vi "Rasnik_SAVE.vi"() -> ()   [LabVIEW 2015]
uses:
  GlobalPath.vi
  Desktop/Mari/GlobalData.vi
panel:
  out "Script":path
  out "Logfile Path":path
  out "Filename selected":path
  out "standard output":string
  out "Y D10":dbl format="%.2f"
  out "Y D9":dbl format="%.2f"
  out "Y D8":dbl format="%.2f"
  out "Y D7":dbl format="%.2f"
  out "Y D6":dbl format="%.2f"
  out "Y D5":dbl format="%.2f"
  out "Y D4":dbl format="%.2f"
  out "Y D3":dbl format="%.2f"
  out "Y D2":dbl format="%.2f"
  out "Y D1":dbl format="%.2f"
  out "X D10":dbl format="%.2f"
  out "X D9":dbl format="%.2f"
  out "X D8":dbl format="%.2f"
  out "X D7":dbl format="%.2f"
  out "X D6":dbl format="%.2f"
  out "X D5":dbl format="%.2f"
  out "X D4":dbl format="%.2f"
  out "X D3":dbl format="%.2f"
  out "X D2":dbl format="%.2f"
  out "X D1":dbl format="%.2f"
  out "Latest file: 2":path
  out "y 6":string
  out "x 6":string
  in  "Done?":bool
  out "y 10":string
  out "x 10":string
  out "y 9":string
  out "x 9":string
  out "y 8":string
  out "x 8":string
  out "y 7":string
  out "x 7":string
  out "y 5":string
  out "x 5":string
  out "y 4":string
  out "x 4":string
  out "y 3":string
  out "x 3":string
  out "y 2":string
  out "x 2":string
  out "y 1":string
  out "x 1":string
  out "Lines":string[](array[string])
  out "Latest file:":path
  in  "Open Program":bool
  in  "c-ccd 3":bool caption="Setup the electronics for the C-CCD reading:\n- make sure the ethernet cables are connected on the minimal heads\n- check that the cable connecting the driver with the mux is plugged in\n- verify that the driver is on and connected to the LAN"
  in  "c-ccd":bool caption="Read the data file"
  # "Rasmask reading from PCBs on stiffback/table"
  # "Run the C-CCD reading program \n(the 10 Rasmasks are automatically read and the data saved)"
  # "Data file reading"
  # "The most recent data file created by the C-CCD program will be opened.\nOnce the \"read data file\" is clicked, the raw data and displacement should appear on the PCB schematics on the bottom."
  # "Displacement (um):"
  # "Raw Data (um):"
  # "Rasmask 1"
  # "Rasmask 2"
  # "Rasmask 1"
  # "Rasmask 2"
  # "Rasmask 3"
  # "Rasmask 4"
  # "Rasmask 3"
  # "Rasmask 4"
  # "Rasmask 6"
  # "Rasmask 5"
  # "Rasmask 6"
  # "Rasmask 5"
  # "Rasmask 7"
  # "Rasmask 8"
  # "Rasmask 7"
  # "Rasmask 8"
  # "Rasmask 9"
  # "Rasmask 10"
  # "Rasmask 9"
  # "Rasmask 10"
  # "Open the DB and load the Rarnik raw file:\nClick on the tab \"RO measurement\" and on the bottom click on \"Load Rasnik 1\" for the table and \"Load  Rasnik 2\" for the stiffback\nLoad the file that appears here --------------------------------------------------------------->\nPress \"SAve info to database\""
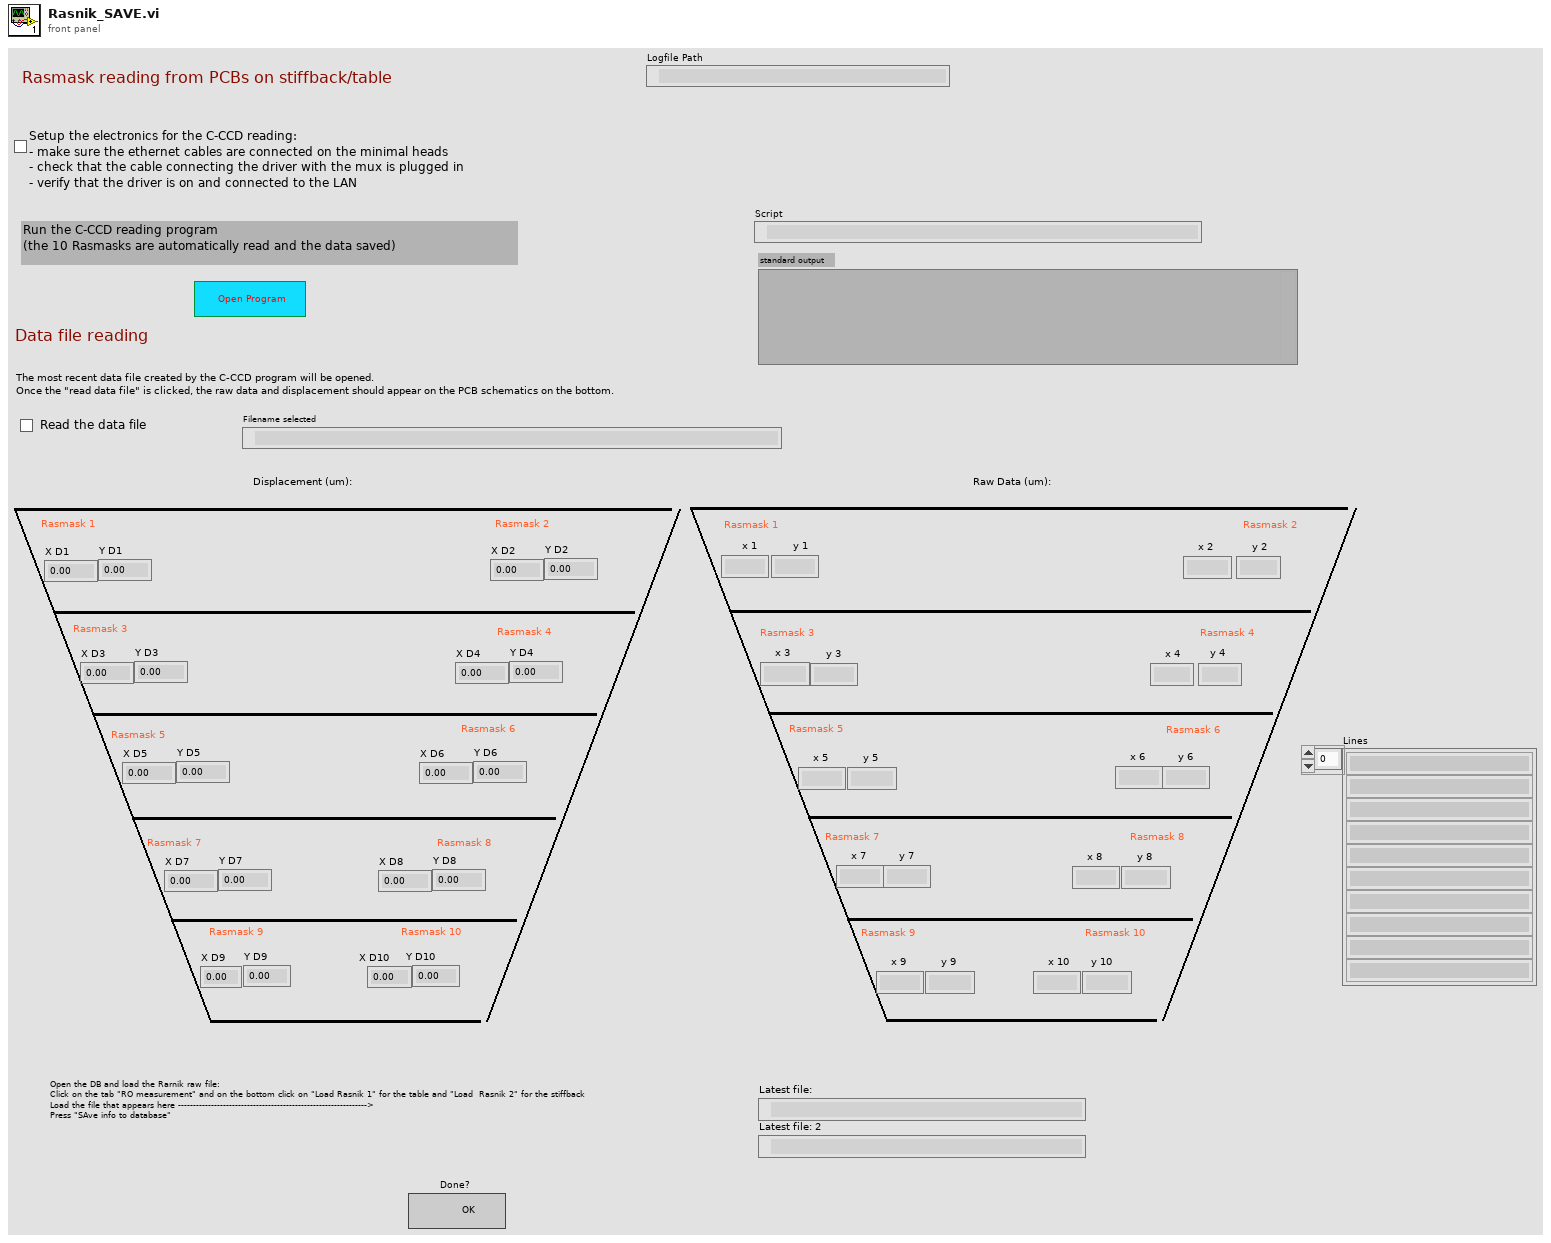
[diagram p1: front panel]
types:
  T1 = enum16{"open", "replace", "create", "open or create", "replace or create", "replace or create with confirmation"}
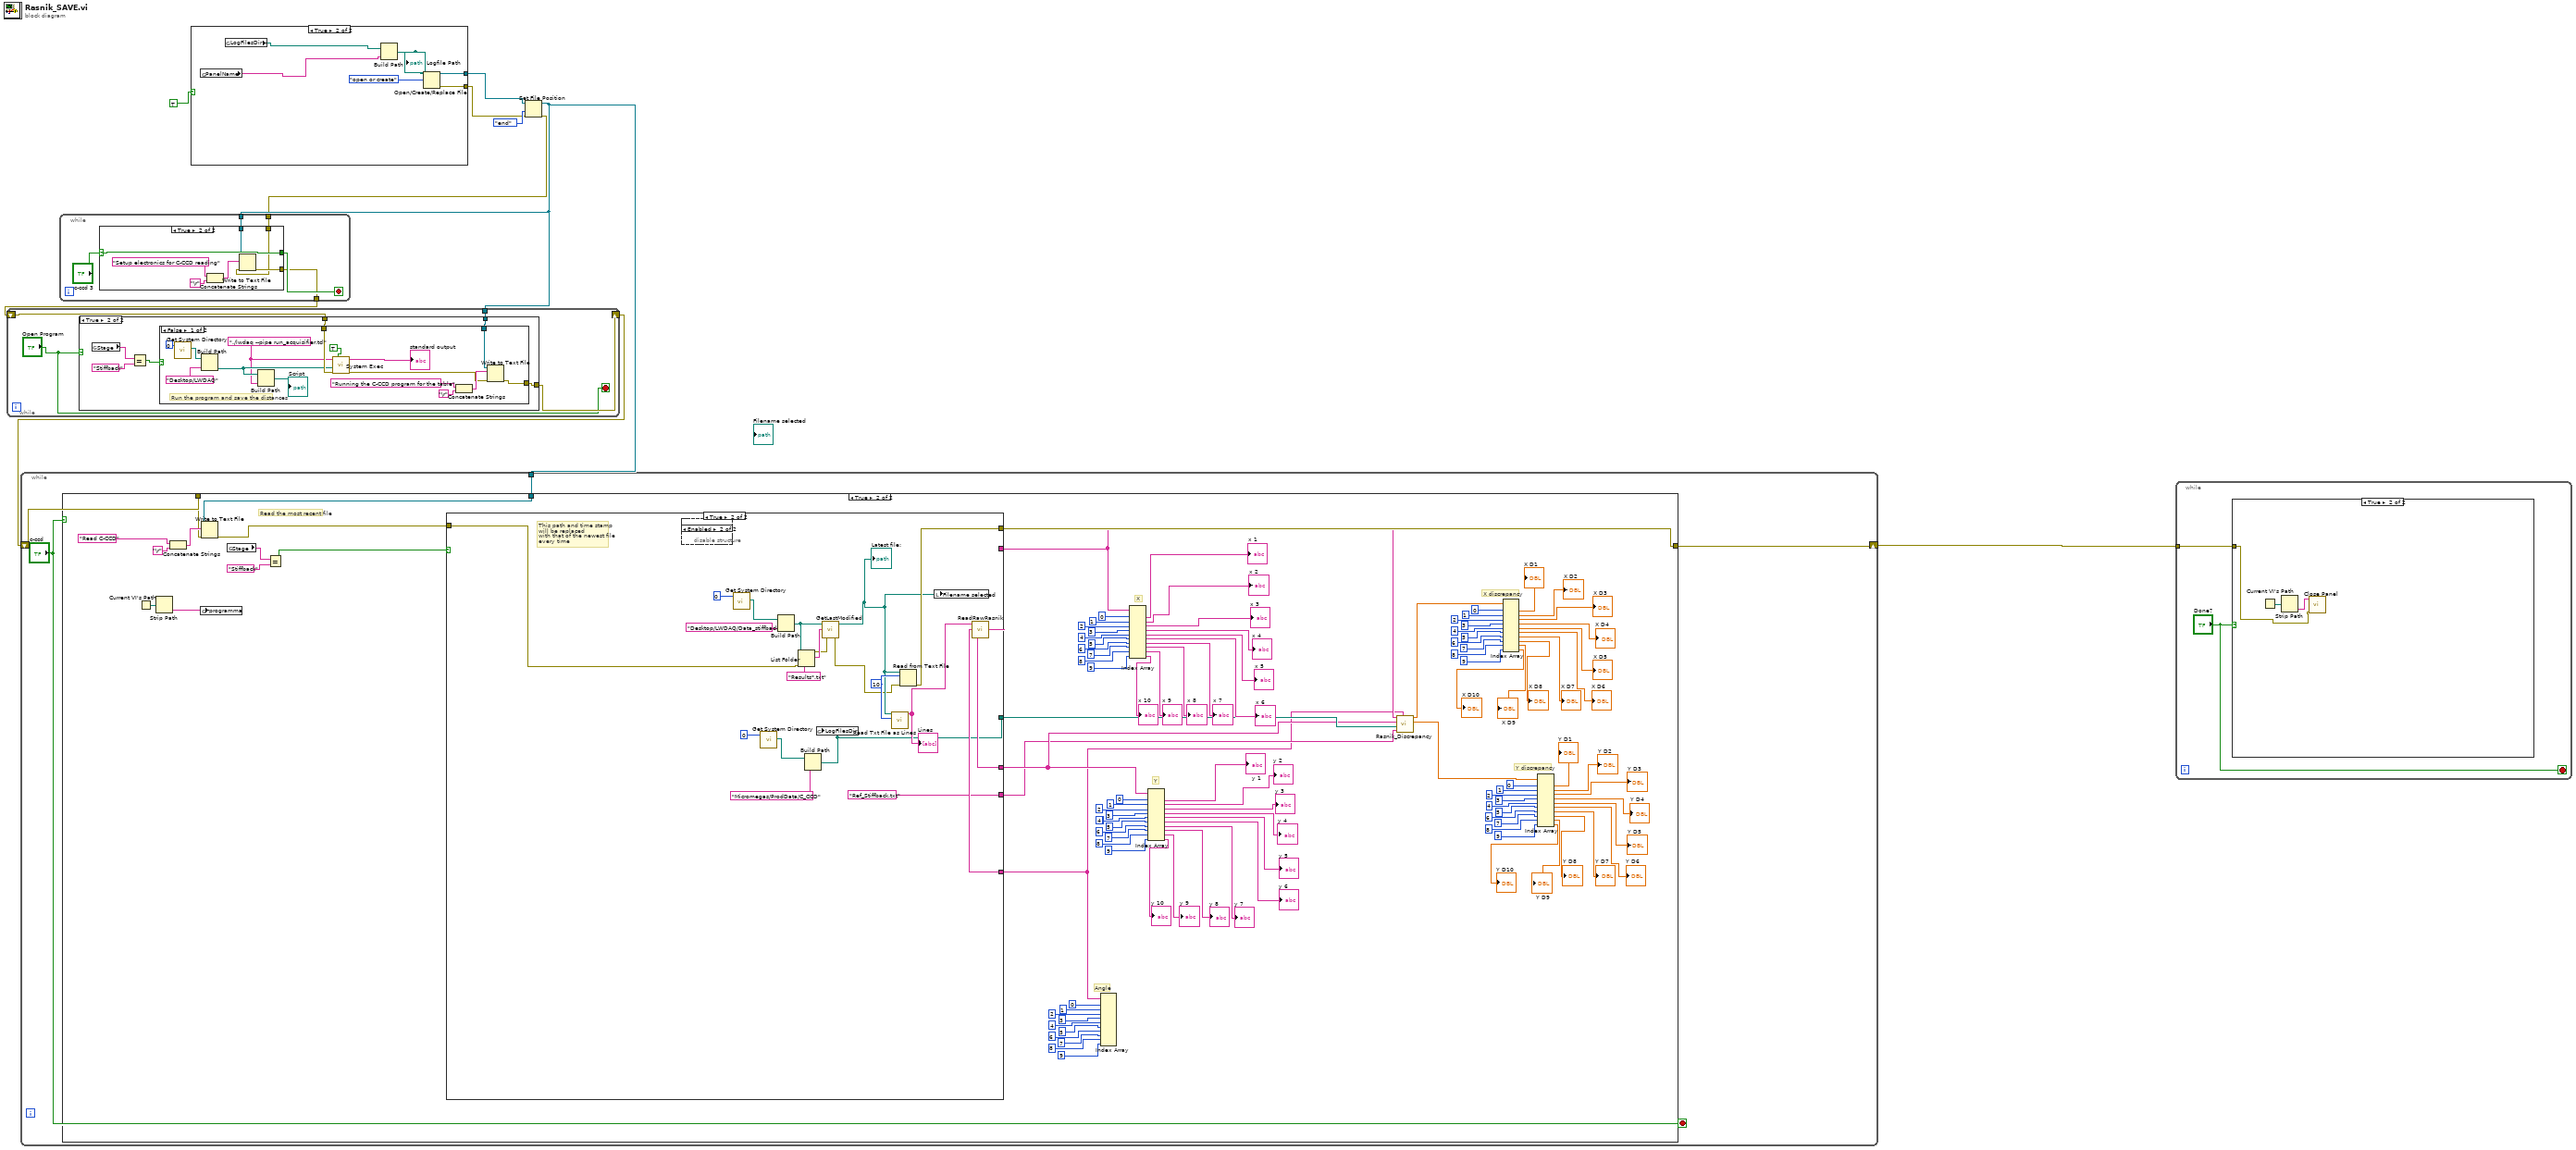
[diagram p0: block diagram]
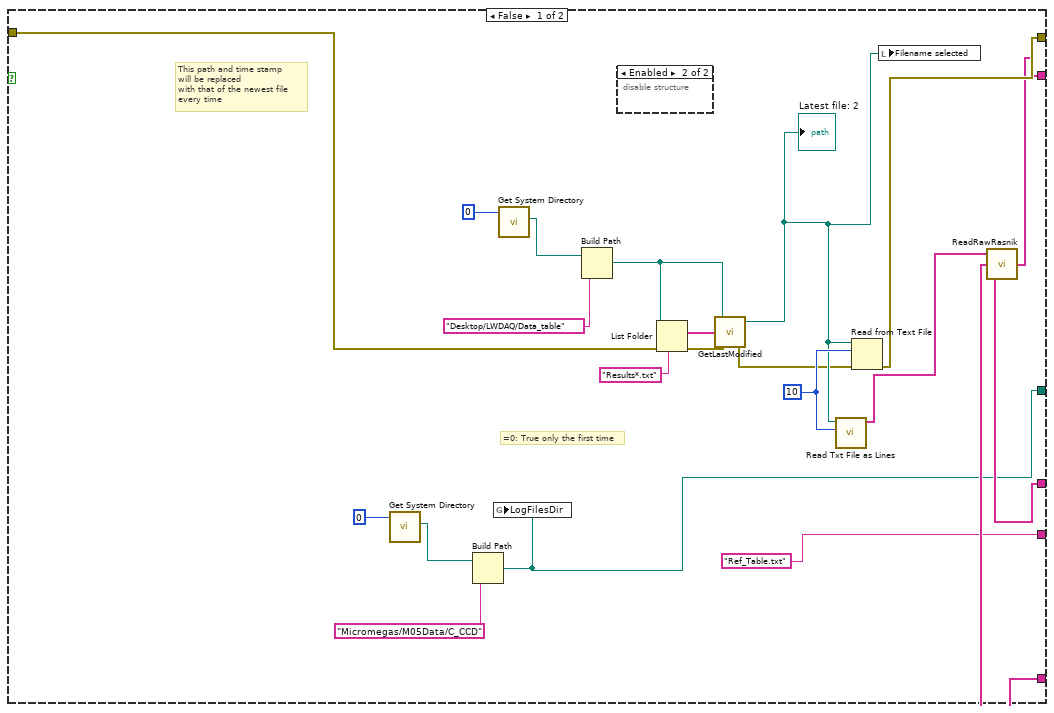
[diagram p4: hidden frame]
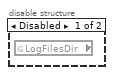
[diagram p5: hidden frame]
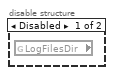
[diagram p6: hidden frame]
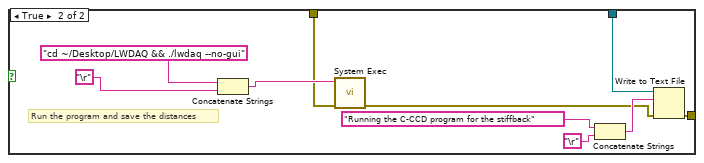
[diagram p9: hidden frame]
diagram:
  n1 = case shown="True" TRUE {
    tunnel: [_ w14] -> w3
    tunnel: [_ w13] -> w4
    frame False {
    }
    frame True {
      n2 = global read "GlobalData.vi" "PanelName"() -> (w10:string)
      n3 = global read "GlobalPath.vi" "LogFilesDir"() -> (w11:path)
      n4 = Build Path(base path=w11, name or relative path=w10) -> (appended path=w15:path)
      "Logfile Path" <- w15
      n5 = Open/Create/Replace File(file path (use dialog)=w15, operation (0:open)=T1."open or create") -> (refnum out=w14:refnum<file>, error out=w13:errorcluster)  [unwired: 4 in, 1 out]
    }
  }
  n6 = Set File Position(refnum=w3, from (0:start)=enum16{"start", "end", "current"}."end", error in=w4) -> (refnum out=w2:refnum<file>, error out=w1:errorcluster)  [unwired: 1 in]
  n7 = while {
    tunnel: w2 -> [w19]
    tunnel: [w17] -> w7
    tunnel: w1 -> [w16]
    stop <- w18 stop-if-true
    n8 = case shown="True" "c-ccd 3" {
      selector: "c-ccd 3" -> [_ w23]
      tunnel: [_ w24] -> w17
      tunnel: w19 -> [_ w21]
      tunnel: [_ w23] -> w18
      tunnel: w16 -> [_ w22]
      frame False {
      }
      frame True {
        n9 = Concatenate Strings("Setup electronics for C-CCD reading", "\r") -> (w27:string)
        n10 = Write to Text File(file (use dialog)=w21, text=w27, error in=w22) -> (error out=w24:errorcluster)  [unwired: 1 in, 2 out]
      }
    }
  }
  n11 = while {
    tunnel: w2 -> [w29]
    shift-right: [w30] -> w9
    shift-left: w7 -> [w31]
    stop <- "Open Program" stop-if-true
    n12 = case shown="True" "Open Program" {
      tunnel: w31 -> [w32 w35]
      tunnel: [w32 w34] -> w30
      tunnel: w29 -> [_ w33]
      frame False {
      }
      frame True {
        n13 = global read "GlobalData.vi" "Stage"() -> (w37:string)
        n14 = Equal?(x=w37, y="Stiffback") -> (x = y?=w36:bool)
        n15 = case shown="False" w36 {
          tunnel: w35 -> [w50 w57]
          tunnel: [w48 w55] -> w34
          tunnel: w33 -> [w47 w54]
          frame False {
            w40 = "./lwdaq --pipe run_acquisifier.tcl"
            # "Run the program and save the distances"
            n16 = call <vilib>:"Get System Directory.vi"("system directory type"=0) -> ("system directory"=w45:path)  [unwired: 10 in]
            n17 = Build Path(base path=w45, name or relative path="Desktop/LWDAQ") -> (appended path=w41:path)
            n18 = Build Path(base path=w41, name or relative path=w40) -> (appended path=→"Script":path)
            n19 = call <vilib>:"System Exec.vi"("wait until completion? (T)"=TRUE, "error in (no error)"=w50, "working directory"=w41, "command line"=w40) -> ("error out"=w49:errorcluster, "standard output"=→"standard output":string)  [unwired: 4 in, 2 out]
            n20 = Concatenate Strings("Running the C-CCD program for the table", "\r") -> (w53:string)
            n21 = Write to Text File(file (use dialog)=w47, text=w53, error in=w49) -> (error out=w48:errorcluster)  [unwired: 1 in, 2 out]
          }
          frame True {
            # "Run the program and save the distances"
            n22 = Concatenate Strings("cd ~/Desktop/LWDAQ && ./lwdaq --no-gui", "\r") -> (w62:string)
            n23 = call <vilib>:"System Exec.vi"("error in (no error)"=w57, "command line"=w62) -> ("error out"=w56:errorcluster)  [unwired: 6 in, 3 out]
            n24 = Concatenate Strings("Running the C-CCD program for the stiffback", "\r") -> (w60:string)
            n25 = Write to Text File(file (use dialog)=w54, text=w60, error in=w56) -> (error out=w55:errorcluster)  [unwired: 1 in, 2 out]
          }
        }
      }
    }
  }
  n26 = while {
    tunnel: w2 -> [w65]
    shift-right: [w66] -> w8
    shift-left: w9 -> [w67]
    stop <- "c-ccd" stop-if-true
    n27 = case shown="True" "c-ccd" {
      tunnel: w67 -> [w68 w169]
      tunnel: [w68 w167] -> w66
      tunnel: w65 -> [_ w166]
      frame False {
      }
      frame True {
        (unwired) 6
        (unwired) 4
        (unwired) 3
        # "Y discrepancy"
        # "X discrepancy"
        # "Angle"
        # "Y"
        # "X"
        # "Read the most recent file"
        n28 = Current VI's Path() -> (path=w170:path)
        n29 = Strip Path(path=w170) -> (name=w171:string)  [unwired: 1 out]
        n30 = Concatenate Strings("Read C-CCD", "\r") -> (w177:string)
        n31 = global write "GlobalData.vi" "programma"(w171) -> ()
        n32 = Write to Text File(file (use dialog)=w166, text=w177, error in=w169) -> (error out=w168:errorcluster)  [unwired: 1 in, 2 out]
        n33 = global read "GlobalData.vi" "Stage"() -> (w173:string)
        n34 = Equal?(x=w173, y="Stiffback") -> (x = y?=w172:bool)
        n35 = case shown="True" w172 {
          tunnel: w168 -> [w178 w199]
          tunnel: [w195 w217] -> w167
          tunnel: [w194 w216] -> w114
          tunnel: [w196 w215] -> w113
          tunnel: [w193 w214] -> w69
          tunnel: [w185 w205] -> w115
          tunnel: ["Ref_Table.txt" "Ref_Stiffback.txt"] -> w112
          frame False {
            w198 = 10
            # "=0: True only the first time"
            # "This path and time stamp\nwill be replaced\nwith that of the newest file \nevery time"
            n36 = call <vilib>:"Get System Directory.vi"("system directory type"=0) -> ("system directory"=w187:path)  [unwired: 10 in]
            n37 = Build Path(base path=w187, name or relative path="Micromegas/M05Data/C_CCD") -> (appended path=w185:path)
            n38 = global write "GlobalPath.vi" "LogFilesDir"(w185) -> ()
            n39 = call <vilib>:"Get System Directory.vi"("system directory type"=0) -> ("system directory"=w190:path)  [unwired: 10 in]
            n40 = Build Path(base path=w190, name or relative path="Desktop/LWDAQ/Data_table") -> (appended path=w180:path)
            n41 = disable-structure shown="Enabled" {
              frame Disabled {
                n42 = global read "GlobalPath.vi" "LogFilesDir"() -> ()  [unwired: 1 out]
              }
              frame Enabled {
              }
            }
            n43 = List Folder(path=w180, pattern="Results*.txt", error in=w178) -> (filenames=w184:string[], error out=w181:errorcluster)  [unwired: 1 in, 2 out]
            n44 = call "GetLastModified.vi"("error in"=w181, "filenames"=w184, "SearchDir"=w180) -> ("error out"=w182:errorcluster, "Path"=w183:path)  [unwired: 1 out]
            "Latest file: 2" <- w183
            n45 = call "Read Txt File as Lines.vi"("Lines to Read"=w198, "file path (use dialog)"=w183) -> ("Lines"=w197:string[])  [unwired: 8 in, 1 out]
            n46 = Read from Text File(file (use dialog)=w183, count=w198, error in=w182) -> (error out=w195:errorcluster)  [unwired: 1 in, 3 out]
            n47 = local write "Filename selected"(w183) -> ()
            n48 = call "ReadRawRasnik.vi"("Lines"=w197) -> ("X cluster"=w194:string[], "Y cluster"=w196:string[], "angle cluster"=w193:string[])
          }
          frame True {
            w219 = 10
            # "This path and time stamp\nwill be replaced\nwith that of the newest file \nevery time"
            n49 = disable-structure shown="Enabled" {
              frame Disabled {
                n50 = global read "GlobalPath.vi" "LogFilesDir"() -> ()  [unwired: 1 out]
              }
              frame Enabled {
              }
            }
            n51 = call <vilib>:"Get System Directory.vi"("system directory type"=0) -> ("system directory"=w211:path)  [unwired: 10 in]
            n52 = call <vilib>:"Get System Directory.vi"("system directory type"=0) -> ("system directory"=w207:path)  [unwired: 10 in]
            n53 = Build Path(base path=w211, name or relative path="Desktop/LWDAQ/Data_stiffback") -> (appended path=w202:path)
            n54 = List Folder(path=w202, pattern="Results*.txt", error in=w199) -> (filenames=w201:string[], error out=w200:errorcluster)  [unwired: 1 in, 2 out]
            n55 = Build Path(base path=w207, name or relative path="Micromegas/ProdData/C_CCD") -> (appended path=w205:path)
            n56 = global write "GlobalPath.vi" "LogFilesDir"(w205) -> ()
            n57 = call "GetLastModified.vi"("error in"=w200, "filenames"=w201, "SearchDir"=w202) -> ("error out"=w203:errorcluster, "Path"=w204:path)  [unwired: 1 out]
            "Latest file:" <- w204
            n58 = call "Read Txt File as Lines.vi"("Lines to Read"=w219, "file path (use dialog)"=w204) -> ("Lines"=w218:string[])  [unwired: 8 in, 1 out]
            "Lines" <- w218
            n59 = Read from Text File(file (use dialog)=w204, count=w219, error in=w203) -> (error out=w217:errorcluster)  [unwired: 1 in, 3 out]
            n60 = local write "Filename selected"(w204) -> ()
            n61 = call "ReadRawRasnik.vi"("Lines"=w218) -> ("X cluster"=w216:string[], "Y cluster"=w215:string[], "angle cluster"=w214:string[])
          }
        }
        n62 = Index Array(array=w69, index #1=0, index #2=1, index #3=2, index #4=3, index #5=4, index #6=5, index #7=6, index #8=7, index #9=8, index #10=9) -> ()  [unwired: 10 out]
        n63 = Index Array(array=w114, index #1=0, index #2=1, index #3=2, index #4=3, index #5=4, index #6=5, index #7=6, index #8=7, index #9=8, index #10=9) -> (element #1=→"x 1":string, element #2=→"x 2":string, element #3=→"x 3":string, element #4=→"x 4":string, element #5=→"x 5":string, element #6=→"x 6":string, element #7=→"x 7":string, element #8=→"x 8":string, element #9=→"x 9":string, element #10=→"x 10":string)
        n64 = Index Array(array=w113, index #1=0, index #2=1, index #3=2, index #4=3, index #5=4, index #6=5, index #7=6, index #8=7, index #9=8, index #10=9) -> (element #1=→"y 1":string, element #2=→"y 2":string, element #3=→"y 3":string, element #4=→"y 4":string, element #5=→"y 5":string, element #6=→"y 6":string, element #7=→"y 7":string, element #8=→"y 8":string, element #9=→"y 9":string, element #10=→"y 10":string)
        n65 = call "Rasnik_Discrepancy.vi"("angle array"=w69, "pattern"=w112, "path"=w115, "Y array"=w113, "X array"=w114) -> ("Y discrepancy"=w71:dbl[], "X discrepancy"=w70:dbl[])  [unwired: 4 in, 1 out]
        n66 = Index Array(array=w70, index #1=0, index #2=1, index #3=2, index #4=3, index #5=4, index #6=5, index #7=6, index #8=7, index #9=8, index #10=9) -> (element #1=→"X D1":dbl, element #2=→"X D2":dbl, element #3=→"X D3":dbl, element #4=→"X D4":dbl, element #5=→"X D5":dbl, element #6=→"X D6":dbl, element #7=→"X D7":dbl, element #8=→"X D8":dbl, element #9=→"X D9":dbl, element #10=→"X D10":dbl)
        n67 = Index Array(array=w71, index #1=0, index #2=1, index #3=2, index #4=3, index #5=4, index #6=5, index #7=6, index #8=7, index #9=8, index #10=9) -> (element #1=→"Y D1":dbl, element #2=→"Y D2":dbl, element #3=→"Y D3":dbl, element #4=→"Y D4":dbl, element #5=→"Y D5":dbl, element #6=→"Y D6":dbl, element #7=→"Y D7":dbl, element #8=→"Y D8":dbl, element #9=→"Y D9":dbl, element #10=→"Y D10":dbl)
      }
    }
  }
  n68 = while {
    tunnel: w8 -> [w221]
    stop <- "Done?" stop-if-true
    n69 = case shown="True" "Done?" {
      tunnel: w221 -> [_ w222]
      frame False {
      }
      frame True {
        n70 = Current VI's Path() -> (path=w223:path)
        n71 = Strip Path(path=w223) -> (name=w224:string)  [unwired: 1 out]
        n72 = call <vilib>:"Close Panel.vi"("error in (no error)"=w222, "VI name"=w224) -> ()  [unwired: 9 in, 1 out]
      }
    }
  }
